vi "OPCUA GetNumberSesssions.vi"(8 "error in (no error)":errorcluster, 10 "handle":u32, 11 "path in":path) -> (0 "error out":errorcluster, 1 "Session Count":i32, 2 "Handle Out":u32, 3 "path out":path)   [LabVIEW 2018]
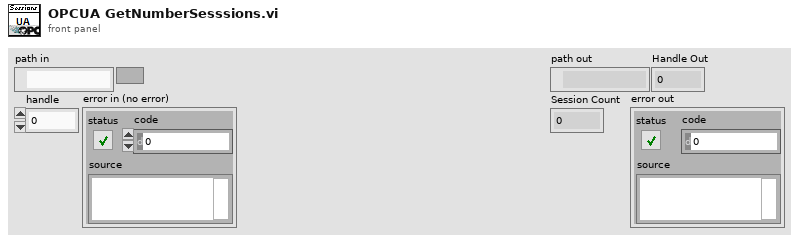
[diagram p1: front panel]
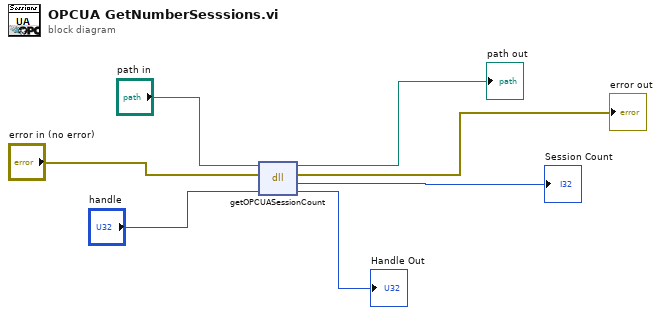
[diagram p0: block diagram]
diagram:
  n1 = dll-call lib="D:/src/HUTCDL/Machine/CDL0100/TagEngine/OPCUA/LVOPCUAInterface.dll" fn="getOPCUASessionCount"(path in="path in", error in="error in (no error)", "handle"="handle") -> (path out=→"path out":path, error out=→"error out":errorcluster, "return type"=→"Session Count":i32, "handle"=→"Handle Out":u32)  [unwired: 1 in]
